vi "GraphViz Generator UI Wrapper.vi"(10 "Modules Configurations":refnum<class "TBM module configuration.lvclass">[](array[class]), 11 "engine configuration in":refnum<class "engine configuration.lvclass">) -> ()   [LabVIEW 2013]
uses:
  <vilib>/NI/Module Execution Interface/Engine Configuration/engine configuration.lvclass
  <vilib>/NI/Tag Bus Module Framework/module configuration/TBM module configuration.lvclass
  System.Drawing
  System.Windows.Forms
  <vilib>/NI/Tag Bus Data Framework/Configuration Editor/Classes/Engine Mappings/Engine Mappings.lvclass
panel:
  in  "GraphViz 'bin' Directory":path=path "C:/Program Files (x86)/Graphviz2.38/bin"
  in  "Zoom?":bool=TRUE
  in  "Tab Control":enum32{"Image", "Modules to Run", "Text"}(tab)
  in  "PictureBox":refnum<k24>(container)
  in  "Modules to View":T1(array[cluster])
  in  "Supported Colors":string[](array[string])=["dodgerblue", "cadetblue1", "darkgoldenrod1", "gainsboro", "palegreen", "peachpuff", "violet", "skyblue", "yellow", "seagreen1", "tomato", "thistle", "slateblue1", "orange", "palevioletred1"]
  out "graphviz data":string
  in  "Close":bool
  in  "Run":bool
  in  "Show Unmapped Channels?":bool=TRUE
  in  "Show Tag Labels?":bool=TRUE
  # "Supported colors list found at \nhttp://www.graphviz.org/doc/info/colors.html"
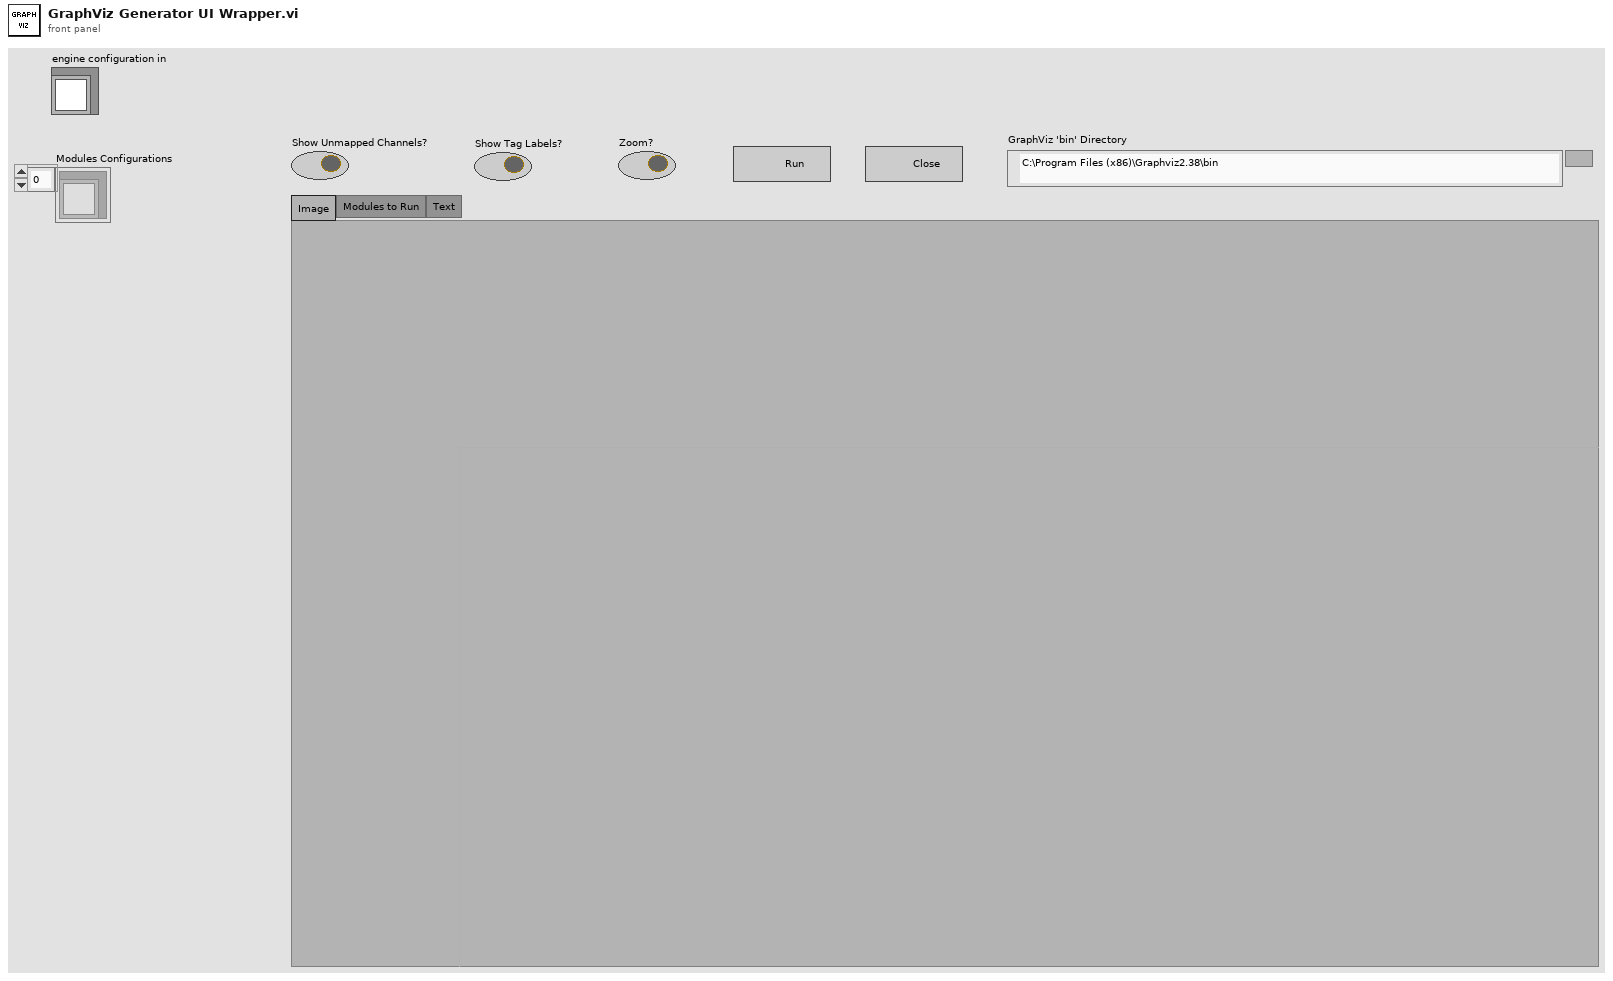
[diagram p1: front panel]
types:
  T1 = cluster{"Module Display Name":string, "View?":bool}[]
  T2 = typedef "PL Framework Configuration Tool.lvlib/Engine Mappings.lvclass/module information.ctl" = cluster{"display name":string, "instance id":string, "channels":refnum<class "TBM channel.lvclass">[]}
  T3 = cluster{"Module Display Name":string, "View?":bool}
  T4 = enum16{"open", "replace", "create", "open or create", "replace or create", "replace or create with confirmation"}
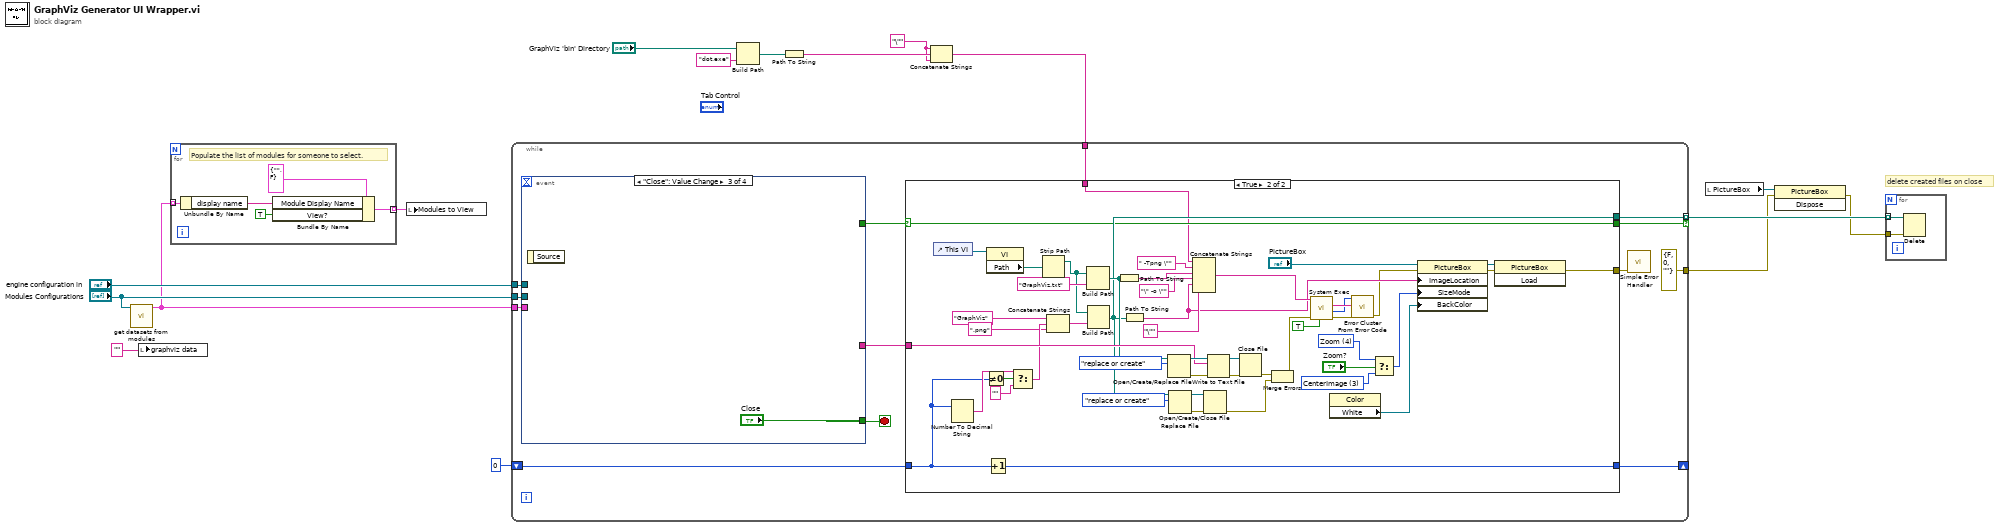
[diagram p0: block diagram]
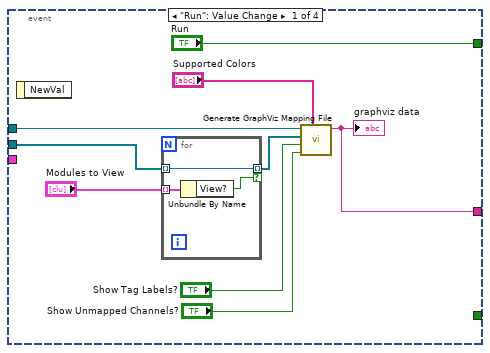
[diagram p3: hidden frame]
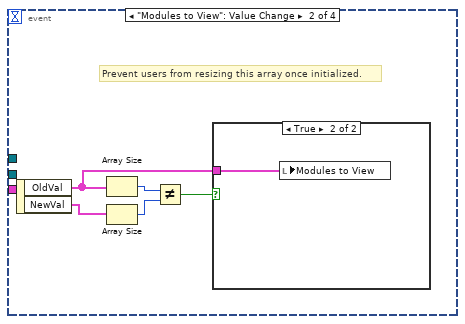
[diagram p4: hidden frame]
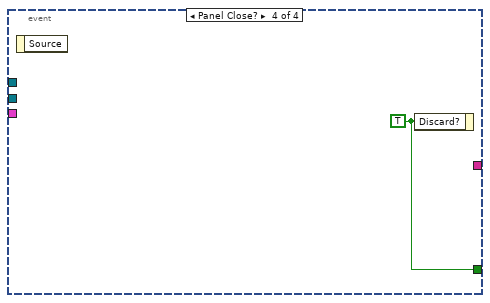
[diagram p6: hidden frame]
diagram:
  w1 = "\"" ("string")
  # "delete created files on close"
  n1 = call <vilib>:"get datasets from modules.vi"("Modules Configurations"="Modules Configurations") -> ("module datasets"=w11:T2[])  [unwired: 9 in, 1 out]
  n2 = local write "graphviz data"("") -> ()
  n3 = for {
    tunnel: w11 -> [w21] mode=indexing
    tunnel: [w17] -> w10 mode=indexing
    # "Populate the list of modules for someone to select."
    n4 = Unbundle By Name(w21) -> ("display name"=w18:string)
    n5 = Bundle By Name(cluster=T3 {"Module Display Name"="", "View?"=FALSE} ("Cluster"), "Module Display Name"=w18, "View?"=TRUE) -> (w17:T3)
  }
  n6 = local write "Modules to View"(w10) -> ()
  n7 = Build Path(base path="GraphViz 'bin' Directory", name or relative path="dot.exe") -> (appended path=w4:path)
  n8 = Path To String(path=w4) -> (string=w5:string)
  n9 = Concatenate Strings(w1, w5, w1) -> (w2:string)
  n10 = while {
    tunnel: "engine configuration in" -> [w34]
    tunnel: "Modules Configurations" -> [w33]
    shift-right: [w29] -> _
    shift-left: 0 -> [w28]
    tunnel: [w27] -> w13 mode=indexing if=w26
    tunnel: w11 -> [w25]
    tunnel: [errorcluster {"status"=FALSE, "code"=0, "source"=""} ("error out")] -> w8
    tunnel: w2 -> [w22]
    stop <- w32 stop-if-true
    n11 = event shown="[2] \"Close\": Value Change" {
      selector: _ -> [_ _ _ _]
      dyn-events: _ -> [_ _ _ _]
      timeout: _ -> [_ _ _ _]
      tunnel: w34 -> [w88 _ _ _]
      tunnel: w33 -> [w87 _ _ _]
      tunnel: [_ _ "Close" w104] -> w32
      tunnel: ["Run" _ _ _] -> w31
      tunnel: [w89 _ _ _] -> w30
      tunnel: w25 -> [_ _ _ _]
      event "Run": Value Change {
        n12 = event-data() -> ()  [unwired: 1 in, 1 out]
        n13 = for {
          tunnel: "Modules to View" -> [w96] mode=indexing
          tunnel: w87 -> [w95] mode=indexing
          tunnel: [w95] -> w86 mode=indexing if=w94
          n14 = Unbundle By Name(w96) -> ("View?"=w94:bool)
        }
        n15 = call "Generate GraphViz Mapping File.vi"("supported colors"="Supported Colors", "Show Unmapped Channels?"="Show Unmapped Channels?", "Show Tag Labels?"="Show Tag Labels?", "Modules Configurations"=w86, "engine configuration in"=w88) -> ("output to graphviz"=w89:string)  [unwired: 6 in]
        "graphviz data" <- w89
      }
      event "Modules to View": Value Change {
        # "Prevent users from resizing this array once initialized."
        n16 = event-data() -> ("OldVal"=w97:T1, "NewVal"=w101:T1)  [unwired: 1 in]
        n17 = Array Size(array=w97) -> (size(s)=w100:i32)
        n18 = Array Size(array=w101) -> (size(s)=w99:i32)
        n19 = Not Equal?(x=w100, y=w99) -> (x != y?=w98:bool)
        n20 = case shown="True" w98 {
          tunnel: w97 -> [_ w102]
          frame False {
          }
          frame True {
            n21 = local write "Modules to View"(w102) -> ()
          }
        }
      }
      event "Close": Value Change {
        n22 = event-data() -> ()  [unwired: 1 in, 1 out]
      }
      event Panel Close? {
        w104 = TRUE ("Discard?")
        n23 = event-data() -> ()  [unwired: 1 in, 1 out]
        n24 = event-data("Discard?"=w104) -> ()  [unwired: 1 in, 1 out]
      }
    }
    n25 = case shown="True" w31 {
      selector: w31 -> [_ w43]
      tunnel: w30 -> [_ w72]
      tunnel: w28 -> [w35 w51]
      tunnel: [w35 w50] -> w29
      tunnel: [_ w44] -> w27
      tunnel: [_ w43] -> w26
      tunnel: [_ w41] -> w24
      tunnel: w22 -> [_ w36]
      frame False {
      }
      frame True {
        w48 = 4 items=["Normal", "StretchImage", "AutoSize", "CenterImage", "Zoom"] ("SizeMode")
        w47 = 3 items=["Normal", "StretchImage", "AutoSize", "CenterImage", "Zoom"] ("SizeMode")
        n26 = control-ref of="This VI"() -> (w78:refnum<vi>)
        n27 = Number To Decimal String(number=w51) -> (decimal integer string=w58:string)  [unwired: 1 in]
        n28 = Not Equal To 0?(x=w51) -> (x != 0?=w59:bool)
        n29 = property class="VI"(reference=w78) -> ("Path"=w79:path)  [unwired: 1 in, 2 out]
        n30 = Increment(x=w51) -> (x+1=w50:i32)
        n31 = Select(t=w58, s=w59, f="") -> (s? t:f=w55:string)
        n32 = Strip Path(path=w79) -> (stripped path=w45:path)  [unwired: 1 out]
        n33 = Concatenate Strings("GraphViz" ("name or relative path"), w55, ".png" ("string")) -> (w53:string)
        n34 = Build Path(base path=w45, name or relative path="GraphViz.txt") -> (appended path=w66:path)
        n35 = Build Path(base path=w45, name or relative path=w53) -> (appended path=w44:path)
        n36 = Path To String(path=w66) -> (string=w81:string)
        n37 = Path To String(path=w44) -> (string=w61:string)
        n38 = Open/Create/Replace File(file path (use dialog)=w66, operation (0:open)=T4."replace or create") -> (refnum out=w73:refnum<file>, error out=w71:errorcluster)  [unwired: 4 in, 1 out]
        n39 = Open/Create/Replace File(file path (use dialog)=w44, operation (0:open)=T4."replace or create") -> (refnum out=w74:refnum<file>, error out=w75:errorcluster)  [unwired: 4 in, 1 out]
        n40 = Concatenate Strings(w36, " -Tpng \"" ("string"), w81, "\" -o \"" ("string"), w61, "\"" ("string")) -> (w65:string)
        n41 = Close File(refnum=w74, error in=w75) -> (error out=w67:errorcluster)  [unwired: 1 out]
        n42 = Write to Text File(file (use dialog)=w73, text=w72, error in=w71) -> (refnum out=w69:refnum<file>, error out=w70:errorcluster)  [unwired: 1 in, 1 out]
        n43 = Close File(refnum=w69, error in=w70) -> (error out=w68:errorcluster)  [unwired: 1 out]
        n44 = Merge Errors(w68, w67) -> (w64:errorcluster)
        n45 = call <vilib>:"System Exec.vi"("run minimized? (F)"=TRUE, "error in (no error)"=w64, "command line"=w65) -> ("error out"=w40:errorcluster, "return code"=w38:i32, "standard error"=w39:string)  [unwired: 5 in, 1 out]
        n46 = property class="Color"() -> ("White"=w52:refnum<k24>)  [unwired: 2 in, 2 out]
        n47 = call <vilib>:"Error Cluster From Error Code.vi"("error in (no error)"=w40, "error message (\"\")"=w39, "error code (0)"=w38) -> ("error out"=w37:errorcluster)  [unwired: 6 in]
        n48 = Select(t=w48, s="Zoom?", f=w47) -> (s? t:f=w46:i32)
        n49 = property class="PictureBox"(reference="PictureBox", error in=w37, "ImageLocation"=w61, "SizeMode"=w46, "BackColor"=w52) -> (reference out=w62:refnum<k24>, error out=w60:errorcluster)
        n50 = invoke class="PictureBox" method="Load"(reference=w62, error in=w60) -> (error out=w41:errorcluster)  [unwired: 1 in, 2 out]
      }
    }
    n51 = call <vilib>:"Simple Error Handler.vi"("error in (no error)"=w24) -> ()  [unwired: 4 in, 5 out]
  }
  n52 = local read "PictureBox"() -> (w9:refnum<k24>)
  n53 = invoke class="PictureBox" method="Dispose"(reference=w9, error in=w8) -> (error out=w7:errorcluster)  [unwired: 1 in, 2 out]
  n54 = for {
    tunnel: w13 -> [w106] mode=indexing
    tunnel: w7 -> [w105]
    n55 = Delete(path (use dialog)=w106, error in=w105) -> ()  [unwired: 3 in, 3 out]
  }
